vi "HEWH UEF Multi.vi"() -> ()   [LabVIEW 2019]
uses:
  Type Definitions/HEWH Water Heater Type.ctl
panel:
  out "error out":errorcluster
  in  "error in (no error)":errorcluster
  in  "Heater Type":T1[](array[typedef])=["Gas Storage (Non-Electric)", "Gas Storage (Non-Electric)", "Standard Electric", "Standard Electric", "Standard Electric", "Standard Electric", "Standard Electric", "Standard Electric", "Standard Electric", "Standard Electric", "Standard Electric", "Standard Electric", "Standard Electric", "Standard Electric", "Standard Electric", "Standard Electric", "Standard Electric", "Standard Electric", "Standard Electric", "Standard Electric", "Standard Electric", "Standard Electric", "Standard Electric", "Standard Electric", "Standard Electric", "Standard Electric", "Standard Electric", "Standard Electric", "Standard Electric", "Standard Electric", "Standard Electric", "Standard Electric", "Standard Electric", "Standard Electric", "Standard Electric", "Standard Electric", "Standard Electric", "Standard Electric", "Standard Electric", "Standard Electric", "Standard Electric", "Standard Electric"]
  out "Numeric":i32
  in  "Volume Array":dbl[](array[numeric])=[38.47, 38.47, 30.07157034, 30.08864439, 30.34664748, 30.03705169, 30.10057558, 30.10057558, 29.94802607, 30.16417656, 29.99194605, 30.04916043, 30.0159685, 29.86419901, 39.90063841, 39.96063937, 39.91740399, 39.84279224, 40.0, 40.0, 39.98847179, 39.99510851, 39.91056187, 39.91392058, 40.0, 39.91056187, 39.83273855, 39.7611926, 39.82508199, 39.70113037, 49.99459193, 50.04505858, 49.78108319, 49.81971154, 50.05041049, 49.87576074, 50.0, 50.00083934, 49.93081875, 49.98317874, 49.77337485, 49.86422512] format="%#.6g"
  in  "Locationi Array":path[](array[path])=[path "C:/TechnologyLab/NI-2010/Trunk/Hybrid Water Heater/Macros/UEF/Example Data/Gas/TR_Rheem 40 gal_Lab_ID_Rheem_Model_XG40T09HE40U0_AmbT__RH__Date_06_02_2020_Time_13_4124 HR_File1_Inv and MC.csv", path "C:/TechnologyLab/NI-2010/Trunk/Hybrid Water Heater/Macros/UEF/Example Data/Gas/TR_Rheem 40 gal_Lab_ID_Rheem_Model_XG40T09HE40U0_AmbT__RH__Date_06_08_2020_Time_09_0824 HR_File0_Inv and MC.csv", path "C:/TechnologyLab/NI-2010/Trunk/Hybrid Water Heater/Macros/UEF/Example Data/Chamber 5/30 Short/19WS1285 30 SHORT BLM 5A UEF Medium.csv", path "C:/TechnologyLab/NI-2010/Trunk/Hybrid Water Heater/Macros/UEF/Example Data/Chamber 5/30 Short/19WS1286 30 SHORT BLM 5A UEF Medium.csv", path "C:/TechnologyLab/NI-2010/Trunk/Hybrid Water Heater/Macros/UEF/Example Data/Chamber 5/30 Short/19WS1287 30 SHORT BLM 5A UEF Med.csv", path "C:/TechnologyLab/NI-2010/Trunk/Hybrid Water Heater/Macros/UEF/Example Data/Chamber 5/30 Short/19WS1288 30 SHORT BLM 5C UEF Med.csv", path "C:/TechnologyLab/NI-2010/Trunk/Hybrid Water Heater/Macros/UEF/Example Data/Chamber 5/30 Short EMV/19WS1261 30 SHORT BMM 5C UEF Medium.csv", path "C:/TechnologyLab/NI-2010/Trunk/Hybrid Water Heater/Macros/UEF/Example Data/Chamber 5/30 Short EMV/19WS1262 30 SHORT BMM 5B UEF Medium.csv", path "C:/TechnologyLab/NI-2010/Trunk/Hybrid Water Heater/Macros/UEF/Example Data/Chamber 5/30 Short EMV/19WS1263 30 SHORT BMM 5B UEF Medium.csv", path "C:/TechnologyLab/NI-2010/Trunk/Hybrid Water Heater/Macros/UEF/Example Data/Chamber 5/30 Short EMV/19WS1264 30 SHORT BMM 5D UEF High X-High.csv", path "C:/TechnologyLab/NI-2010/Trunk/Hybrid Water Heater/Macros/UEF/Example Data/Chamber 5/30 Tall/19WS1273 30 TALL BLM 5D UEF Medium.csv", path "C:/TechnologyLab/NI-2010/Trunk/Hybrid Water Heater/Macros/UEF/Example Data/Chamber 5/30 Tall/19WS1274 30 TALL BLM 5C UEF Medium.csv", path "C:/TechnologyLab/NI-2010/Trunk/Hybrid Water Heater/Macros/UEF/Example Data/Chamber 5/30 Tall/19WS1275 30 TALL BLM 5D UEF Medium.csv", path "C:/TechnologyLab/NI-2010/Trunk/Hybrid Water Heater/Macros/UEF/Example Data/Chamber 5/30 Tall/19WS1276 30 TALL BLM 5D UEF Med.csv", path "C:/TechnologyLab/NI-2010/Trunk/Hybrid Water Heater/Macros/UEF/Example Data/Chamber 5/40 Short/19WS1281 40 SHORT BLM 5B UEF Medium.csv", path "C:/TechnologyLab/NI-2010/Trunk/Hybrid Water Heater/Macros/UEF/Example Data/Chamber 5/40 Short/19WS1282 40 SHORT BLM 5C UEF Medium.csv", path "C:/TechnologyLab/NI-2010/Trunk/Hybrid Water Heater/Macros/UEF/Example Data/Chamber 5/40 Short/19WS1283 40 SHORT BLM 5C UEF Medium.csv", path "C:/TechnologyLab/NI-2010/Trunk/Hybrid Water Heater/Macros/UEF/Example Data/Chamber 5/40 Short/19WS1284 40 SHORT BLM 5B UEF Med.csv", path "C:/TechnologyLab/NI-2010/Trunk/Hybrid Water Heater/Macros/UEF/Example Data/Chamber 5/40 Short EMV/19WS1257 40 SHORT BMM 5A UEF Medium Manual EMV.csv", path "C:/TechnologyLab/NI-2010/Trunk/Hybrid Water Heater/Macros/UEF/Example Data/Chamber 5/40 Short EMV/19WS1258 40 SHORT BMM 5D UEF Medium Manual EMV.csv", path "C:/TechnologyLab/NI-2010/Trunk/Hybrid Water Heater/Macros/UEF/Example Data/Chamber 5/40 Short EMV/19WS1259 40 SHORT BMM 5B UEF Med v6.10.1.35 Production PS 122F.csv", path "C:/TechnologyLab/NI-2010/Trunk/Hybrid Water Heater/Macros/UEF/Example Data/Chamber 5/40 Short EMV/19WS1260 40 SHORT BMM 5B UEF Med v6.10.1.35 Production PS 122F.csv", path "C:/TechnologyLab/NI-2010/Trunk/Hybrid Water Heater/Macros/UEF/Example Data/Chamber 5/40 Tall/19WS1269 40 TALL BLM 5B UEF Medium 122F.csv", path "C:/TechnologyLab/NI-2010/Trunk/Hybrid Water Heater/Macros/UEF/Example Data/Chamber 5/40 Tall/19WS1270 40 TALL BLM 5D UEF Medium 122F.csv", path "C:/TechnologyLab/NI-2010/Trunk/Hybrid Water Heater/Macros/UEF/Example Data/Chamber 5/40 Tall/19WS1271 40 TALL BLM 5D UEF Medium 122F Extra UE Insulation.csv", path "C:/TechnologyLab/NI-2010/Trunk/Hybrid Water Heater/Macros/UEF/Example Data/Chamber 5/40 Tall/19WS1272 40 TALL BLM 5A UEF Medium 122F Extra UE Insulation2.csv", path "C:/TechnologyLab/NI-2010/Trunk/Hybrid Water Heater/Macros/UEF/Example Data/Chamber 5/40 Tall/20WS1026 40 TALL BLM 5A UEF Med 122F.csv", path "C:/TechnologyLab/NI-2010/Trunk/Hybrid Water Heater/Macros/UEF/Example Data/Chamber 5/40 Tall/20WS1027 40 TALL BLM 5B UEF Med 123F.csv", path "C:/TechnologyLab/NI-2010/Trunk/Hybrid Water Heater/Macros/UEF/Example Data/Chamber 5/40 Tall/20WS1028 40 TALL BLM 5C UEF Med 123F.csv", path "C:/TechnologyLab/NI-2010/Trunk/Hybrid Water Heater/Macros/UEF/Example Data/Chamber 5/40 Tall/20WS1029 40 TALL BLM 5D UEF Med 122F.csv", path "C:/TechnologyLab/NI-2010/Trunk/Hybrid Water Heater/Macros/UEF/Example Data/Chamber 5/50 Short/19WS1277 50 SHORT BLM 5C UEF High.csv", path "C:/TechnologyLab/NI-2010/Trunk/Hybrid Water Heater/Macros/UEF/Example Data/Chamber 5/50 Short/19WS1278 50 SHORT BLM 5B UEF High.csv", path "C:/TechnologyLab/NI-2010/Trunk/Hybrid Water Heater/Macros/UEF/Example Data/Chamber 5/50 Short/19WS1279 50 SHORT BLM 5D UEF High.csv", path "C:/TechnologyLab/NI-2010/Trunk/Hybrid Water Heater/Macros/UEF/Example Data/Chamber 5/50 Short/19WS1280 50 SHORT BLM 5C UEF High.csv", path "C:/TechnologyLab/NI-2010/Trunk/Hybrid Water Heater/Macros/UEF/Example Data/Chamber 5/50 Short EMV/19WS1253 50 SHORT BMM 5B UEF High v6.5.93.25.csv", path "C:/TechnologyLab/NI-2010/Trunk/Hybrid Water Heater/Macros/UEF/Example Data/Chamber 5/50 Short EMV/19WS1254 50 SHORT BMM 5C UEF High v6.5.92.25.csv", path "C:/TechnologyLab/NI-2010/Trunk/Hybrid Water Heater/Macros/UEF/Example Data/Chamber 5/50 Short EMV/19WS1255 50 SHORT BMM 5B UEF High UE Opt v6.10.1.35.csv", path "C:/TechnologyLab/NI-2010/Trunk/Hybrid Water Heater/Macros/UEF/Example Data/Chamber 5/50 Short EMV/19WS1256 50 SHORT BMM 5B UEF High X-High.csv", path "C:/TechnologyLab/NI-2010/Trunk/Hybrid Water Heater/Macros/UEF/Example Data/Chamber 5/50 Tall/19WS1265 50 TALL BLM 5B UEF High.csv", path "C:/TechnologyLab/NI-2010/Trunk/Hybrid Water Heater/Macros/UEF/Example Data/Chamber 5/50 Tall/19WS1266 50 TALL BLM 5C UEF High.csv", path "C:/TechnologyLab/NI-2010/Trunk/Hybrid Water Heater/Macros/UEF/Example Data/Chamber 5/50 Tall/19WS1267 50 TALL BLM 5A UEF High.csv", path "C:/TechnologyLab/NI-2010/Trunk/Hybrid Water Heater/Macros/UEF/Example Data/Chamber 5/50 Tall/19WS1268 50 TALL BLM 5A UEF High.csv"]
  out "transposed array":string[][](array[string])
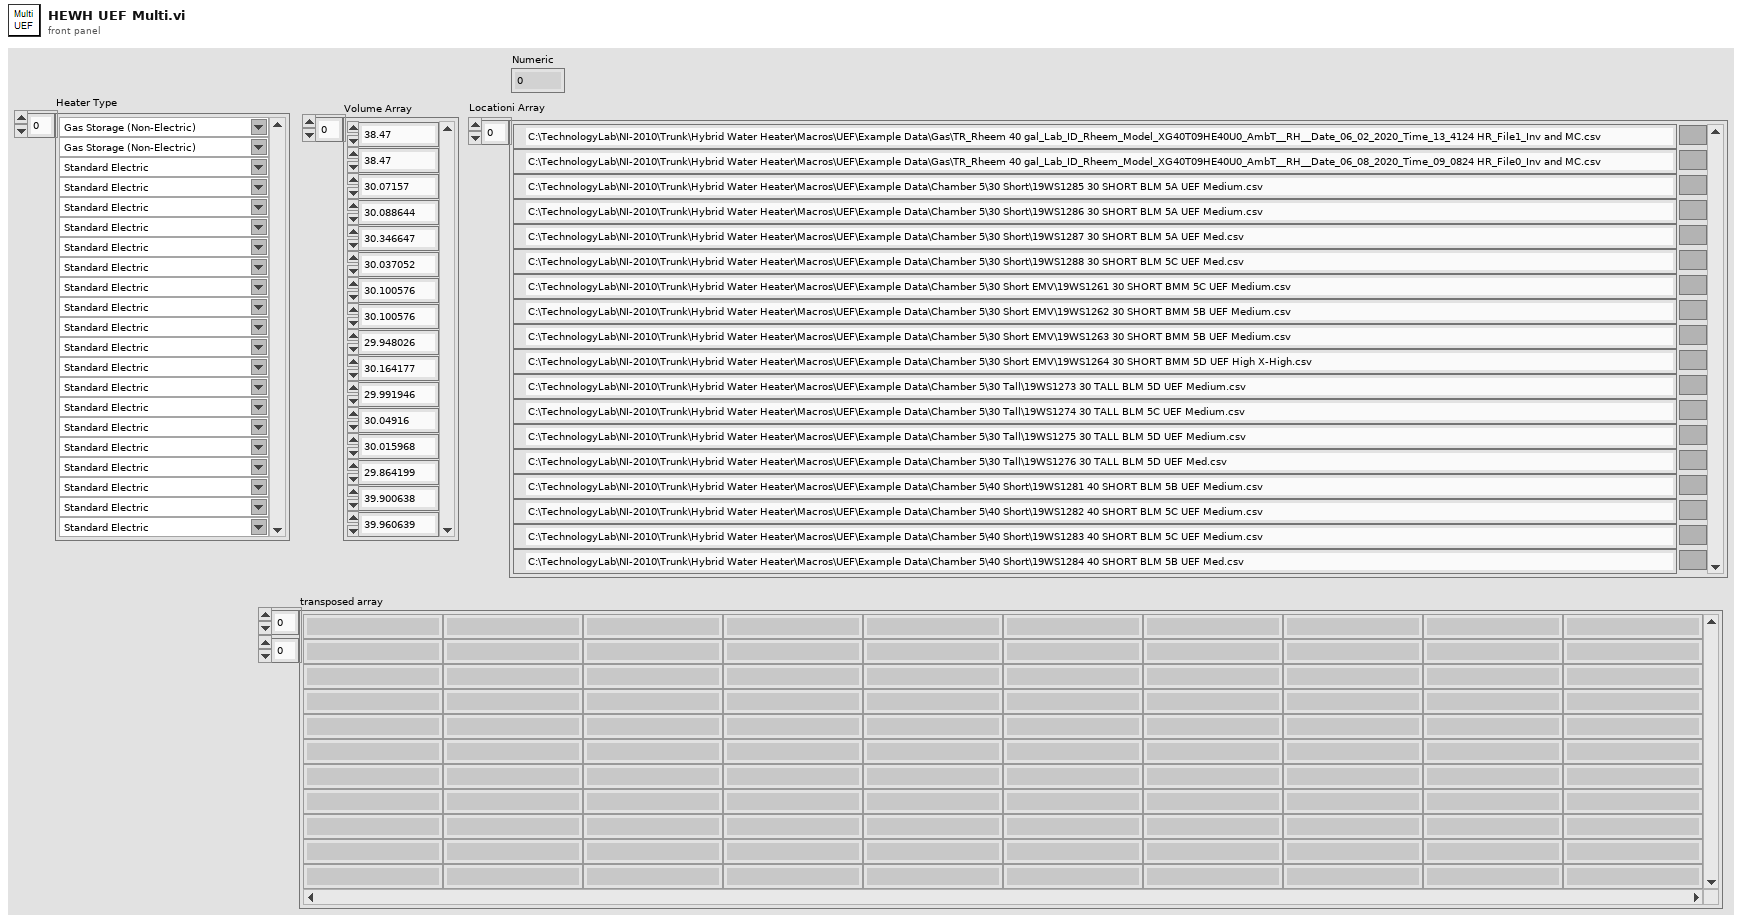
[diagram p1: front panel]
types:
  T1 = typedef "HEWH Water Heater Type.ctl" = string
  T2 = typedef "UEF Constants.ctl" = cluster{"Calculated Values":T3, "Sampled Data":cluster{"Cold Water Draw Amounts-(Gal)":dbl[], "T del_all - Outlet Temps (°F)":dbl[], "T in_all - Inlet Temps (°F)":dbl[], "Qsu0 (BTU)":dbl, "Qsuf (BTU)":dbl, "Tau stby_1 (hr)":dbl, "T suf(°F)":dbl, "T su0(°F)":dbl, "T tstby(°F)":dbl, "T astby(°F)":dbl, "T 24(°F)":dbl, "Qr (BTU)":dbl, "T0 (°F)":dbl, "Tmax1 (°F)":dbl, "Qe (BTU)":dbl, "Qf (BTU)":dbl, "Tastby2 (°F)":dbl, "RTD Out Full Data Set (Each Draw)":dbl[][], "RTD IN Full Data Set (Each Draw)":dbl[][], "Tau stby2 (hr)":dbl, "Hot Water Draw Amounts-(Gal)":dbl[], "Cold Flow Rate (GPM)":dbl[][], "Hot Flow Rate (GPM)":dbl[][]}, "Static Data":cluster{"T-Wh Setpoint (°F)":dbl, "T-Inlet Setpoint (°F)":dbl, "T-Ambinet Nominal (°F)":dbl, "V - Volume of Wh (True)":dbl}, "Data Indexes":cluster{"Test Start Index  (Full Index)":i32, "Header Length":i32, "Draw Index":i32[][], "Tmax1 Recovery Draw #":i32, "Start Watt Hours":dbl, "Tsu0 Index":i32, "Tsf Index":i32, "Start Energy (BTU-Gas)":dbl, "Usage Cluster":T4, "T0 Index (Full Data Index)":i32, "Non-Draw Index":i32[][], "Tmax1 Index":i32, "Test End Index  (Full Index)":i32, "Heating Index":i32[][], "Heating Timestamp":dbl[][], "Non-Draw Timestamp":dbl[][], "Draw Index Timestamp":dbl[][], "Tmax1 Timestamp":dbl, "Tsu0 Timestamp":dbl, "Tsf Timestamp":dbl, "T0 Timestamp":dbl, "Test End Timestamp":dbl, "Test Start Timestamp":dbl, "5 sec after Draw Index\nTemp (Avg)":dbl[][]}, "Raw Data":cluster{"Elapsed Time Index":i32, "Software Elapsed Time Index":i32, "TC Tree Avg Index":i32, "Watt Hours (Wh) Index":i32, "Energy (BTU) Index":i32, "Totalized Flow Index":i32, "Flow Rate Index":i32, "Program Status Index":i32, "RTDin Index":i32, "RTDout Index":i32, "RTDamb Index":i32, "Test Data-Start to End DBL":dbl[][], "Data Type":T5, "Heat Source Index":i32, "Hot Water Rate (GPM)":i32, "Hot Water Total (gal)":i32}, "Tolerance Check (T)=Pass":cluster{"Flow Rate":bool, "Totalized Flow":bool, "Ambient Temp":bool, "Ambient Humidity":bool, "Inlet Temp":bool, "Outlet Temp":bool, "Valid Test":bool, "Individual Totalized Flow":bool, "Data Sheet Check":string}}
  T3 = typedef "HEWH Draw Stats.ctl" = cluster{"Draw Cluster - Actual (Gal)":dbl[], "Mass of water All (lbm)":dbl[], "Density of hot water All (lbm/gal)":dbl[], "CpHW (BTU/(lbm °F))":dbl[], "rho 2 (lb/gal)":dbl, "rho standby (lb/gal)":dbl, "rho 24 (lb/gal)":dbl, "Cp1 (BTU/(lb*F))":dbl, "Cp2 (BTU/(lb*F))":dbl, "Cp standby (BTU/(lb*F))":dbl, "Cp 24 (BTU/(lb*F))":dbl, "nu_r":dbl, "Qstby (BTU)":dbl, "Qhr (BTU/hr)":dbl, "UA (BTU/(hr*F))":dbl, "Q (BTU)":dbl, "Qd (BTU)":dbl, "Qda (BTU)":dbl, "QHW67 (BTU)":dbl, "UEF":dbl, "Tdel1 - Mean Outlet 1st Cluster (°F)":dbl, "Tin1 - Mean Inlet 1st Cluster (°F)":dbl, "Cp theoretical (BTU/(lbm °F))":dbl, "M cluster mass removed (lb)":dbl, "V1- Vol (Gal)":dbl, "Test Data -Start to End":string[][], "rho_nu (lb/gal)":dbl, "Density of cold water All (lbm/gal)":dbl[], "CpUEF (BTU/(lb*F))":dbl, "QHW (BTU)":dbl, "QHWD (BTU)":dbl, "Qdm (BTU)":dbl}
  T4 = typedef "HEWH Usage Cluster.ctl" = string
  T5 = typedef "HEWH Meter Type.ctl" = enum16{"GEA Inlet Side Meter", "GEA Outlet Side Meter", "CSA Inlet Side Meter"}
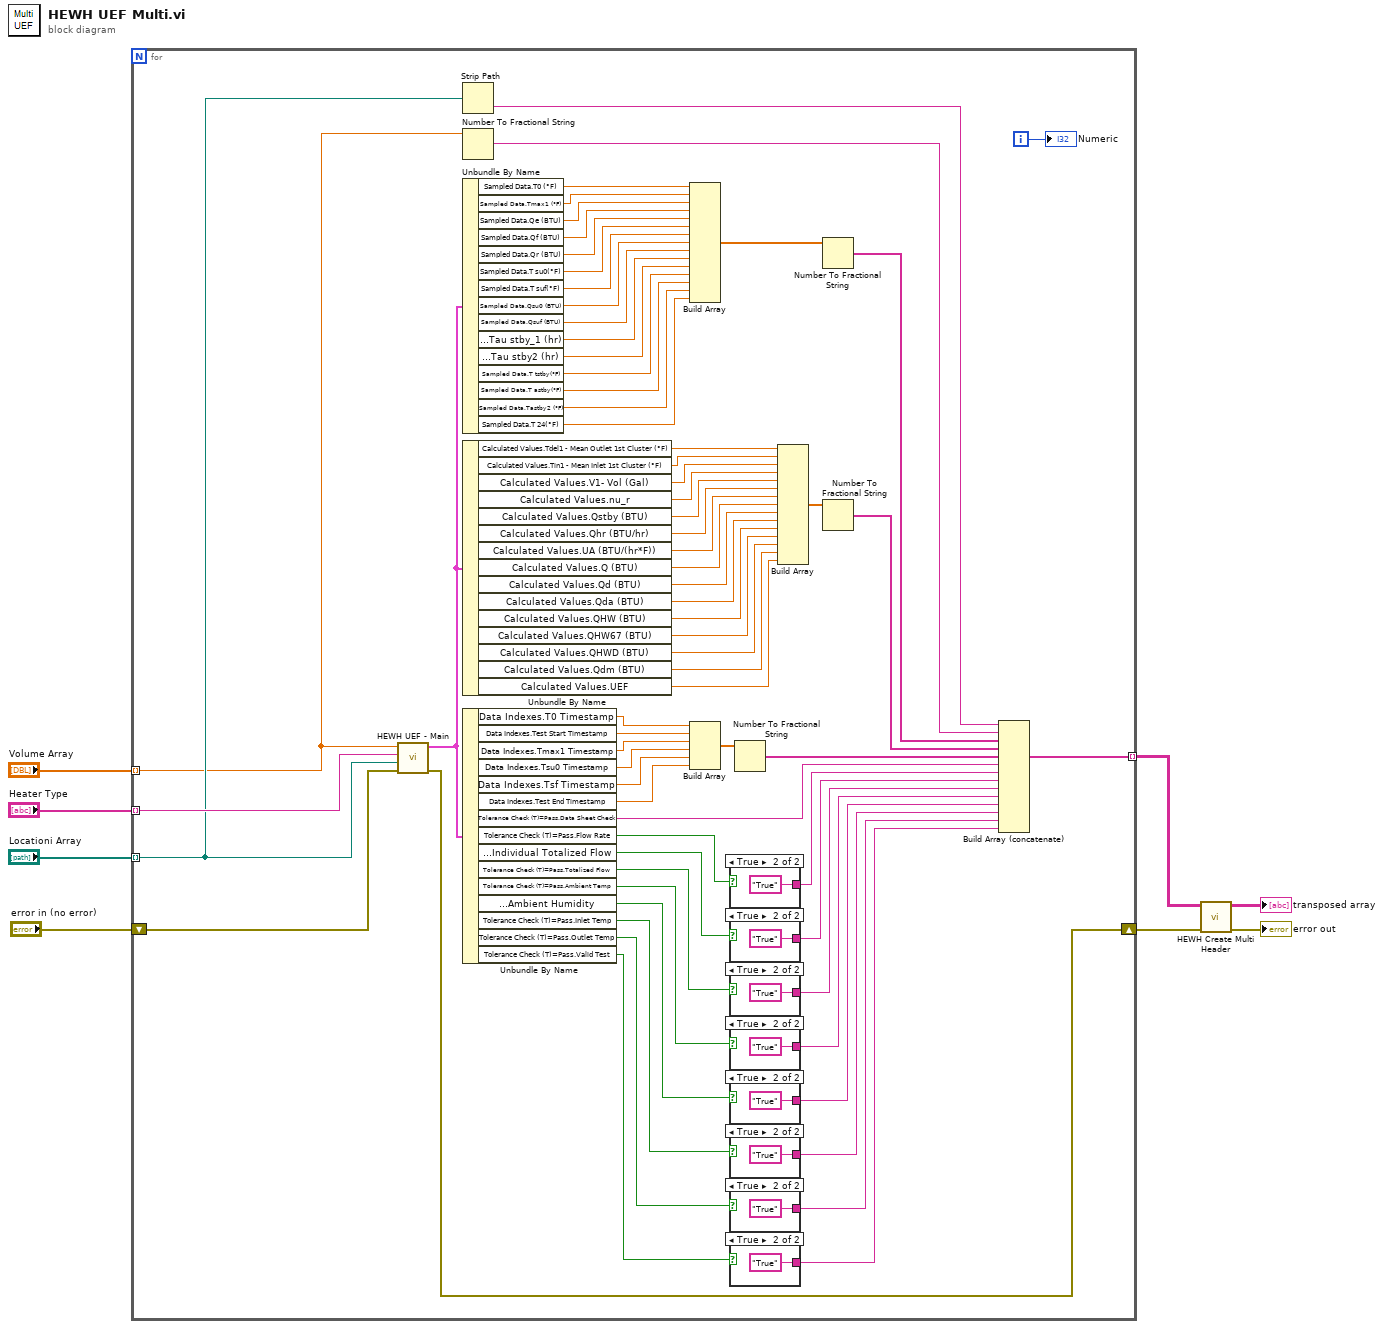
[diagram p0: block diagram]
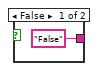
[diagram p2: hidden frame]
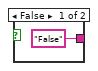
[diagram p3: hidden frame]
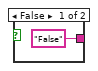
[diagram p4: hidden frame]
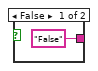
[diagram p5: hidden frame]
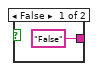
[diagram p6: hidden frame]
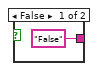
[diagram p7: hidden frame]
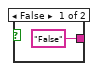
[diagram p8: hidden frame]
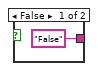
[diagram p9: hidden frame]
diagram:
  n1 = for {
    tunnel: "Heater Type" -> [w70] mode=indexing
    tunnel: "Locationi Array" -> [w12] mode=indexing
    tunnel: [w67] -> w8 mode=indexing
    tunnel: "Volume Array" -> [w11] mode=indexing
    shift-right: [w13] -> w2
    shift-left: "error in (no error)" -> [w14]
    i -> [w69]
    n2 = call "HEWH UEF - Main.vi"("Error In"=w14, "file path (dialog if empty)"=w12, "Water Heater Type"=w70, "True Tank Capacity"=w11) -> ("Error Out"=w13:errorcluster, "UEF Calculated Values Output"=w49:T2)  [unwired: 6 in]
    n3 = Strip Path(path=w12) -> (name=w10:string)  [unwired: 1 out]
    n4 = Number To Fractional String(number=w11) -> (F-format string=w9:string)  [unwired: 3 in]
    n5 = Unbundle By Name(w49) -> ("Sampled Data.T0 (°F)"=w46:dbl, "Sampled Data.Tmax1 (°F)"=w45:dbl, "Sampled Data.Qe (BTU)"=w44:dbl, "Sampled Data.Qf (BTU)"=w43:dbl, "Sampled Data.Qr (BTU)"=w42:dbl, "Sampled Data.T su0(°F)"=w41:dbl, "Sampled Data.T suf(°F)"=w40:dbl, "Sampled Data.Qsu0 (BTU)"=w39:dbl, "Sampled Data.Qsuf (BTU)"=w38:dbl, "Sampled Data.Tau stby_1 (hr)"=w37:dbl, "Sampled Data.Tau stby2 (hr)"=w36:dbl, "Sampled Data.T tstby(°F)"=w35:dbl, "Sampled Data.T astby(°F)"=w34:dbl, "Sampled Data.Tastby2 (°F)"=w33:dbl, "Sampled Data.T 24(°F)"=w32:dbl)
    n6 = Unbundle By Name(w49) -> ("Calculated Values.Tdel1 - Mean Outlet 1st Cluster (°F)"=w31:dbl, "Calculated Values.Tin1 - Mean Inlet 1st Cluster (°F)"=w30:dbl, "Calculated Values.V1- Vol (Gal)"=w29:dbl, "Calculated Values.nu_r"=w28:dbl, "Calculated Values.Qstby (BTU)"=w27:dbl, "Calculated Values.Qhr (BTU/hr)"=w26:dbl, "Calculated Values.UA (BTU/(hr*F))"=w25:dbl, "Calculated Values.Q (BTU)"=w24:dbl, "Calculated Values.Qd (BTU)"=w23:dbl, "Calculated Values.Qda (BTU)"=w22:dbl, "Calculated Values.QHW (BTU)"=w21:dbl, "Calculated Values.QHW67 (BTU)"=w20:dbl, "Calculated Values.QHWD (BTU)"=w19:dbl, "Calculated Values.Qdm (BTU)"=w18:dbl, "Calculated Values.UEF"=w17:dbl)
    n7 = Unbundle By Name(w49) -> ("Data Indexes.T0 Timestamp"=w77:dbl, "Data Indexes.Test Start Timestamp"=w76:dbl, "Data Indexes.Tmax1 Timestamp"=w75:dbl, "Data Indexes.Tsu0 Timestamp"=w74:dbl, "Data Indexes.Tsf Timestamp"=w73:dbl, "Data Indexes.Test End Timestamp"=w72:dbl, "Tolerance Check (T)=Pass.Data Sheet Check"=w66:string, "Tolerance Check (T)=Pass.Flow Rate"=w65:bool, "Tolerance Check (T)=Pass.Individual Totalized Flow"=w64:bool, "Tolerance Check (T)=Pass.Totalized Flow"=w63:bool, "Tolerance Check (T)=Pass.Ambient Temp"=w62:bool, "Tolerance Check (T)=Pass.Ambient Humidity"=w61:bool, "Tolerance Check (T)=Pass.Inlet Temp"=w60:bool, "Tolerance Check (T)=Pass.Outlet Temp"=w59:bool, "Tolerance Check (T)=Pass.Valid Test"=w58:bool)
    n8 = Build Array(w46, w45, w44, w43, w42, w41, w40, w39, w38, w37, w36, w35, w34, w33, w32) -> (w47:dbl[])
    n9 = Build Array(w77, w76, w75, w74, w73, w72) -> (w71:dbl[])
    n10 = case shown="True" w65 {
      tunnel: ["False" "True"] -> w57
      frame False {
      }
      frame True {
      }
    }
    n11 = case shown="True" w64 {
      tunnel: ["False" "True"] -> w56
      frame False {
      }
      frame True {
      }
    }
    n12 = case shown="True" w63 {
      tunnel: ["False" "True"] -> w55
      frame False {
      }
      frame True {
      }
    }
    n13 = case shown="True" w62 {
      tunnel: ["False" "True"] -> w54
      frame False {
      }
      frame True {
      }
    }
    n14 = case shown="True" w61 {
      tunnel: ["False" "True"] -> w53
      frame False {
      }
      frame True {
      }
    }
    n15 = case shown="True" w60 {
      tunnel: ["False" "True"] -> w52
      frame False {
      }
      frame True {
      }
    }
    n16 = case shown="True" w59 {
      tunnel: ["False" "True"] -> w51
      frame False {
      }
      frame True {
      }
    }
    n17 = case shown="True" w58 {
      tunnel: ["False" "True"] -> w50
      frame False {
      }
      frame True {
      }
    }
    n18 = Number To Fractional String(number=w71) -> (F-format string=w68:string[])  [unwired: 3 in]
    n19 = Build Array(w31, w30, w29, w28, w27, w26, w25, w24, w23, w22, w21, w20, w19, w18, w17) -> (w48:dbl[])
    n20 = Number To Fractional String(number=w47) -> (F-format string=w15:string[])  [unwired: 3 in]
    n21 = Number To Fractional String(number=w48) -> (F-format string=w16:string[])  [unwired: 3 in]
    n22 = Build Array (concatenate)(w10, w9, w15, w16, w68, w66, w57, w56, w55, w54, w53, w52, w51, w50) -> (w67:string[])
    "Numeric" <- w69
  }
  n23 = call "HEWH Create Multi Header.vi"("error in (no error)"=w2, "Array in"=w8) -> ("error out"=→"error out":errorcluster, "Array out"=→"transposed array":string[][])  [unwired: 8 in]
